vi "uAssembler_Call.vi"(0 "Path":path) -> ()   [LabVIEW 2021, in "uFramework_pack_uActor.lvlib" / "uAssembler.lvclass"]
doc: "To use this VI, use a \"call-by-reference\" node in the caller VI and pass in the lvclass filepath.\nThe caller shall not be statically linked to any classes. It is meant to be a lightweight splashscreen without any dependencies.\n\nWhere needed, use a special queue named 'splash' to report the progress in loading classes without creating a static dependency between the caller and the callee."
uses:
  uAssembler.lvclass
  Bin/uFramework.lvlibp/uTransport_uActor/uTransport_uActor.lvclass
  uAssembler.lvclass/uAssembler.ctl
  Bin/uFramework.lvlibp/uActor/uActor.lvclass
  U:/Projects/uFramework/Bin/uFramework.lvlibp/uActor/uActor.lvclass
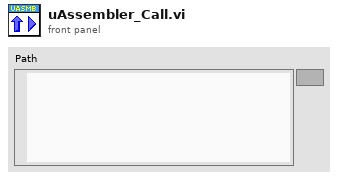
[diagram p1: front panel]
types:
  T1 = enum32{"invalid app kind", "Development System", "Run Time System", "Student Edition", "Embedded LabVIEW", "Evaluation", "Custom"}
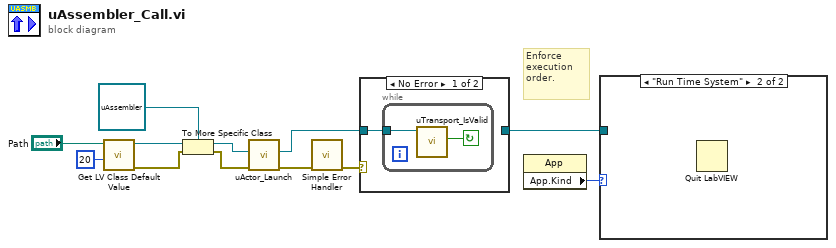
[diagram p0: block diagram]
diagram:
  # "Enforce execution order."
  n1 = call <vilib>:"Get LV Class Default Value.vi"("options"=u32 20, "class path"="Path") -> ("error out"=w7:errorcluster, "object"=w10:refnum<class>)  [unwired: 8 in]
  n2 = To More Specific Class(target class=refnum<class "uAssembler.lvclass"> refnum ("uAssembler.lvlib:uAssembler.lvclass"), reference=w10, error in=w7) -> (specific class reference=w2:refnum<class "uAssembler.lvclass">, error out=w3:errorcluster)
  n3 = call "uActor_Launch.vi"("error in (no error)"=w3, "Actor to Launch"=w2) -> ("error out"=w1:errorcluster, "uTransport_uActor"=w12:refnum<class "uTransport_uActor.lvclass">)  [unwired: 7 in, 1 out]
  n4 = call <vilib>:"Simple Error Handler.vi"("error in (no error)"=w1) -> ("error out"=w11:errorcluster)  [unwired: 4 in, 4 out]
  n5 = case shown="No Error" w11 {
    tunnel: w12 -> [w13 w16]
    tunnel: [_ w16] -> w4
    frame No Error {
      n6 = while {
        tunnel: w13 -> [w14]
        stop <- w15 continue-if-true
        n7 = call-dynamic "uTransport_IsValid.vi"("uTransport_uActor in"=w14) -> ("IsValid?"=w15:bool)  [unwired: 8 in, 2 out]
      }
    }
    frame Error {
    }
  }
  n8 = property class="App"() -> ("App.Kind"=w5:T1)  [unwired: 2 in, 2 out]
  n9 = case shown="\"Run Time System\"" w5 {
    tunnel: w4 -> [_ _]
    frame Default {
    }
    frame "Run Time System" {
      n10 = Quit LabVIEW() -> ()  [unwired: 1 in]
    }
  }
